vi "周期设置_总磷总氮.vi"() -> ()   [LabVIEW 2016, in "斯坦道氨氮.lvlib"]
uses:
  <vilib>/Utility/miscctls.llb/LVPointTypeDef.ctl
  <vilib>/Utility/config.llb/NI_LVConfig.lvlib
panel:
  in  "运行周期":T1={"运行模式"=enum."维护模式", "质控频次"=enum."关闭", "空白核查时间"=2, "跨度核查时间"=6, "24H周期设置"=[]} {"跨度核查时间" items=["00H", "01H", "02H", "03H", "04H", "05H", "06H", "07H", "08H", "09H", "10H", "11H", "12H", "13H", "14H", "15H", "16H", "17H", "18H", "19H", "20H", "21H", "22H", "23H", "关闭"]; "空白核查时间" items=["00H", "01H", "02H", "03H", "04H", "05H", "06H", "07H", "08H", "09H", "10H", "11H", "12H", "13H", "14H", "15H", "16H", "17H", "18H", "19H", "20H", "21H", "22H", "23H", "关闭"]}
  # "运行模式："
  # "质控频次："
  # "零点核查时间："
  # "跨度核查时间："
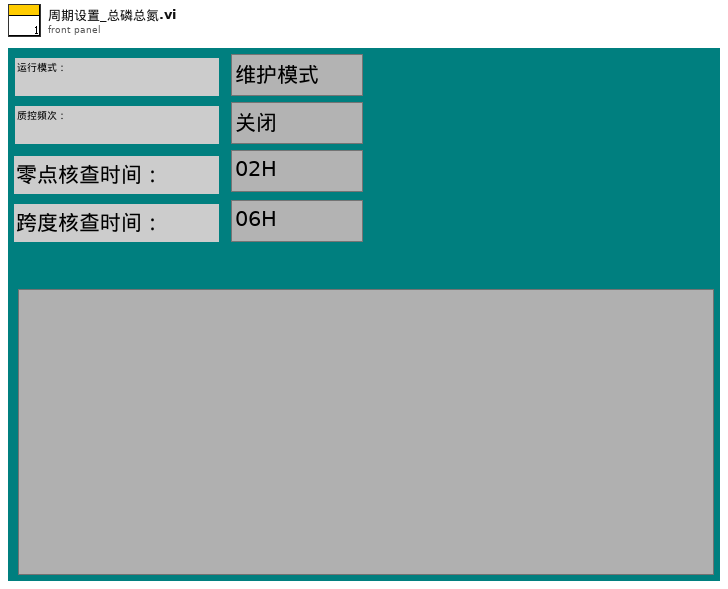
[diagram p1: front panel]
types:
  T1 = cluster{"运行模式":enum16{"维护模式", "常规模式", "应急模式", "质控模式"}, "质控频次":enum16{"关闭", "每天", "星期一", "星期二", "星期三", "星期四", "星期五", "星期六", "星期日"}, "空白核查时间":u16, "跨度核查时间":u16, "24H周期设置":bool[]}
  T2 = typedef "LVPointTypeDef.ctl" = cluster{"Horizontal":i16, "Vertical":i16}
  T3 = enum16{"启动测量", "标样核查", "零点核查", "跨度核查", "空白测试", "平行样测试", "加标回收", "空白校准", "标样校准", "初始化（清洗）", "停止测试", "仪器重启", "校时", "模式设置", "测量间隔设置"}
  T4 = cluster{"系统时间":timestamp, "工作状态":enum16{"空闲", "水样测试", "标样核查", "零点核查", "跨度核查", "空白测试", "平行样测试", "加标回收", "空白校准", "标样校准", "初始化（清洗）"}, "测量模式":enum16{"待机", "连续模式", "周期模式", "定点模式", "受控模式", "手动模式"}, "告警代码":u16, "故障代码":u16, "日志代码":u16, "软件版本":u16, "F0":sgl, "F1":sgl, "F2":sgl, "F3":sgl, "T":sgl, "H":sgl, "id":u16, "flowid":u16, "量程":u16, "总磷控温温度1":sgl, "营养盐控温温度2":sgl, "ADC":sgl}
  T5 = enum16{"关闭", "每天", "星期一", "星期二", "星期三", "星期四", "星期五", "星期六", "星期日"}
  T6 = typedef "LVDateTimeRec.ctl" = cluster{"秒数的小数部分":dbl, "秒":i32, "分":i32, "时":i32, "日":i32, "月":i32, "年":i32, "天数（周）":i32, "天数（年）":i32, "DST":i32}
  T7 = enum32{"Bad", "Idle", "Run top level", "Running"}
  T8 = typedef "NI_LVConfig.lvlib/Config Data RefNum.ctl" = refnum<k1>
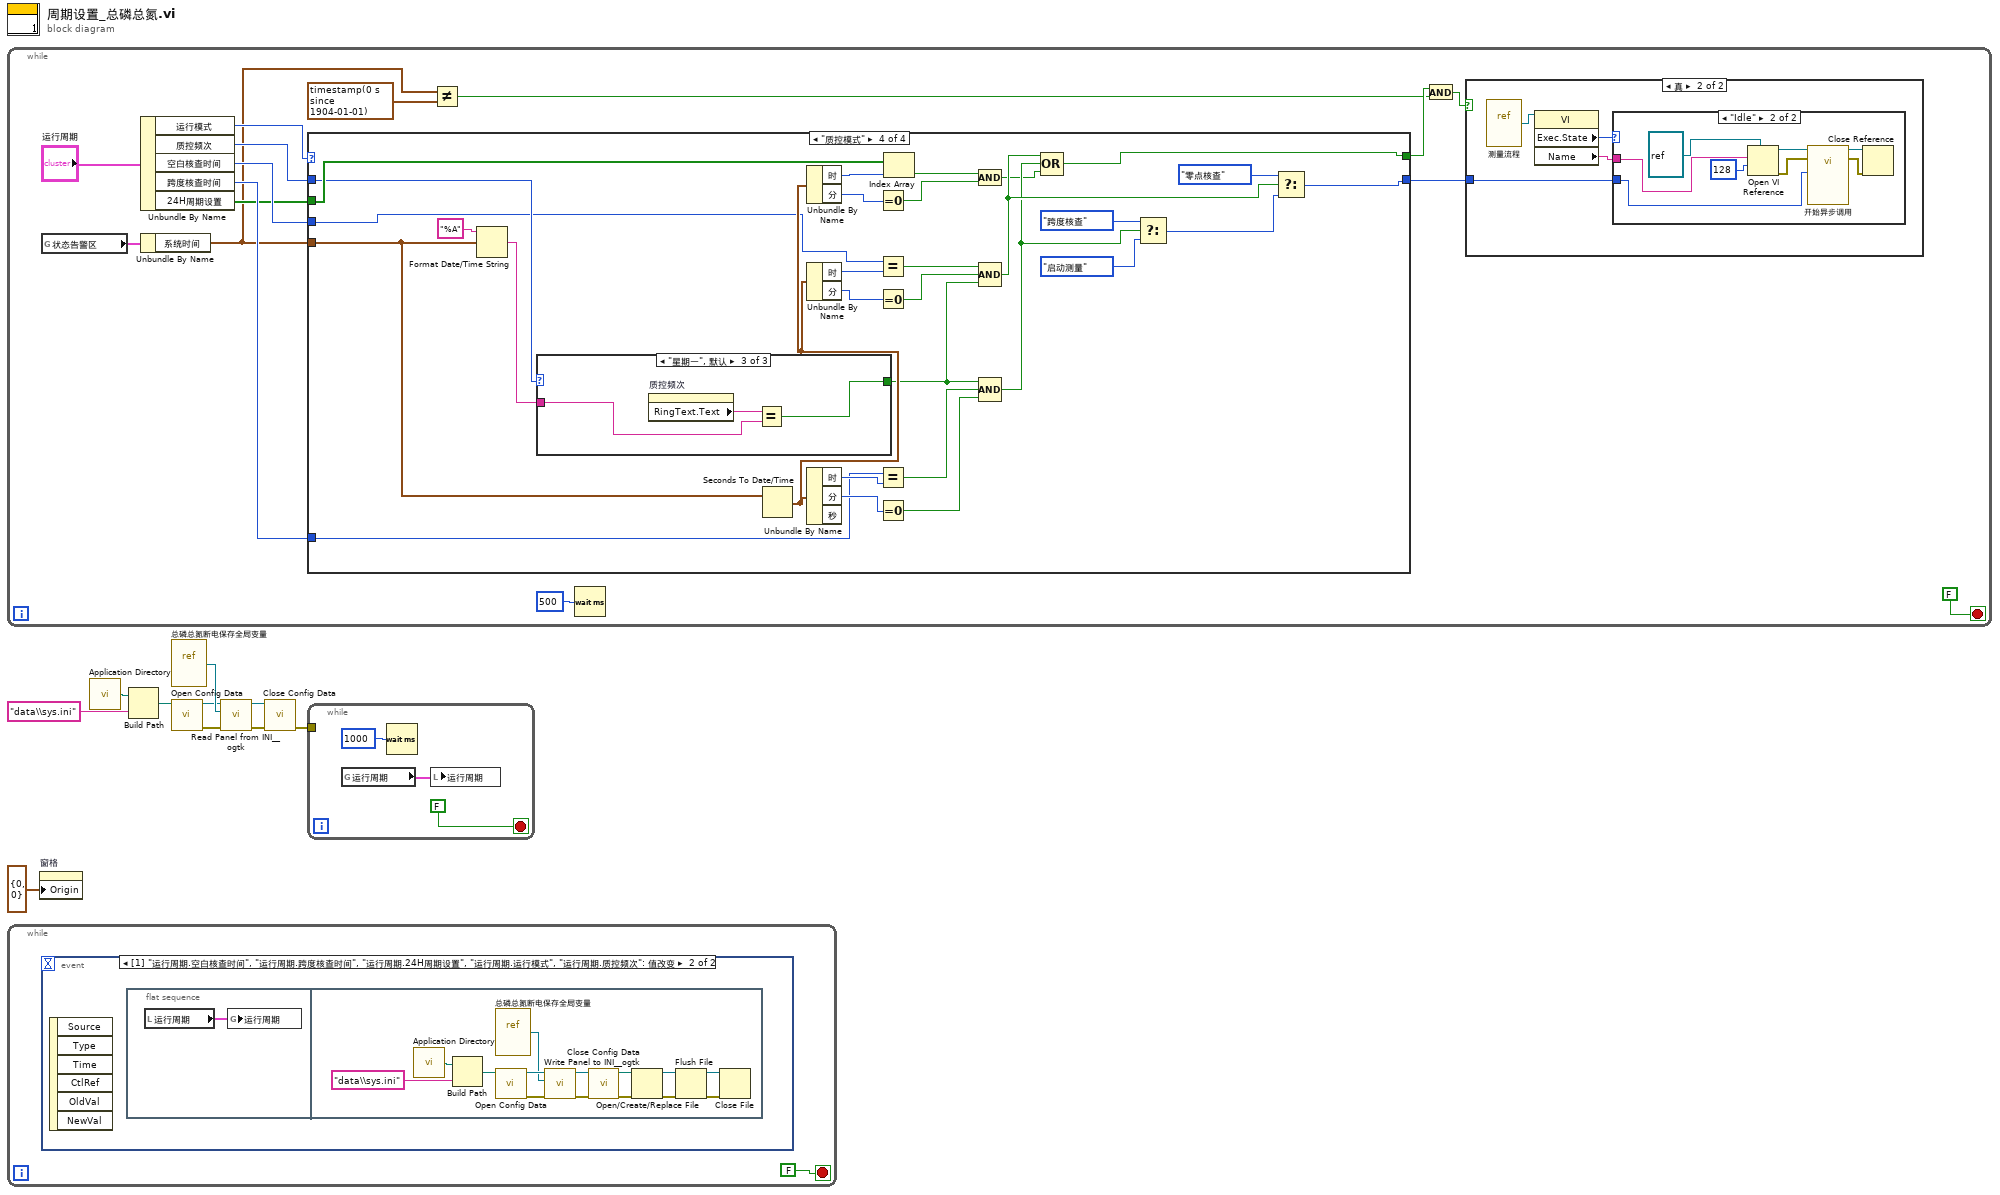
[diagram p0: block diagram]
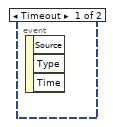
[diagram p2: hidden frame]
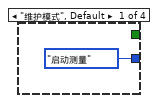
[diagram p5: hidden frame]
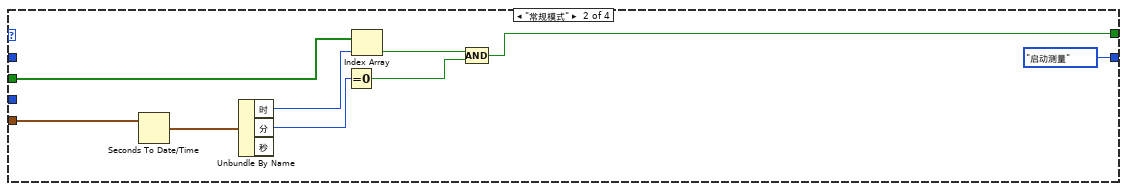
[diagram p6: hidden frame]
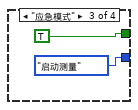
[diagram p7: hidden frame]
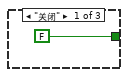
[diagram p8: hidden frame]
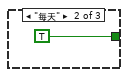
[diagram p9: hidden frame]
diagram:
  n1 = while {
    stop <- FALSE stop-if-true
    n2 = global read "VAR总磷总氮全局变量.vi" "状态告警区"() -> (w15:T4)
    n3 = Unbundle By Name("运行周期") -> ("运行模式"=w22:enum16{"维护模式", "常规模式", "应急模式", "质控模式"}, "质控频次"=w21:T5, "空白核查时间"=w20:u16, "跨度核查时间"=w19:u16, "24H周期设置"=w18:bool[])
    n4 = Unbundle By Name(w15) -> ("系统时间"=w14:timestamp)
    n5 = case shown="\"质控模式\"" w22 {
      tunnel: w14 -> [_ w47 _ w79]
      tunnel: w18 -> [_ w44 _ w76]
      tunnel: [_ w40 TRUE w62] -> w17
      tunnel: [T3."启动测量" ("控制命令") T3."启动测量" ("控制命令") T3."启动测量" ("控制命令") w58] -> w16
      tunnel: w21 -> [_ _ _ w55]
      tunnel: w20 -> [_ _ _ w54]
      tunnel: w19 -> [_ _ _ w53]
      frame "维护模式", Default {
      }
      frame "常规模式" {
        n6 = Seconds To Date/Time(time stamp (now)=w47) -> (date time rec=w46:T6)  [unwired: 1 in]
        n7 = Unbundle By Name(w46) -> ("时"=w45:i32, "分"=w43:i32)  [unwired: 1 out]
        n8 = Equal To 0?(x=w43) -> (x = 0?=w41:bool)
        n9 = Index Array(array=w44, index=w45) -> (element=w42:bool)
        n10 = Compound Arithmetic op=AND ("复合运算")(w42, w41) -> (w40:bool)
      }
      frame "应急模式" {
      }
      frame "质控模式" {
        n11 = Format Date/Time String(time format string (%c)="%A" ("时间格式字符串(%c)"), seconds (now)=w79) -> (date/time string=w77:string)  [unwired: 1 in]
        n12 = case shown="\"星期一\", 默认" w55 {
          tunnel: w77 -> [_ _ w83]
          tunnel: [FALSE TRUE w82] -> w56
          frame "关闭" {
          }
          frame "每天" {
          }
          frame "星期一", Default {
            n13 = property on="质控频次" class="Enum (严格)"() -> ("RingText.Text"=w84:string)  [unwired: 2 in, 2 out]
            n14 = Equal?(x=w84, y=w83) -> (x = y?=w82:bool)
          }
        }
        n15 = Seconds To Date/Time(time stamp (now)=w79) -> (date time rec=w65:T6)  [unwired: 1 in]
        n16 = Unbundle By Name(w65) -> ("时"=w75:i32, "分"=w73:i32)
        n17 = Unbundle By Name(w65) -> ("时"=w71:i32, "分"=w70:i32)
        n18 = Unbundle By Name(w65) -> ("时"=w66:i32, "分"=w67:i32)  [unwired: 1 out]
        n19 = Equal To 0?(x=w73) -> (x = 0?=w72:bool)
        n20 = Equal?(x=w54, y=w71) -> (x = y?=w69:bool)
        n21 = Equal To 0?(x=w70) -> (x = 0?=w68:bool)
        n22 = Equal?(x=w53, y=w66) -> (x = y?=w64:bool)
        n23 = Equal To 0?(x=w67) -> (x = 0?=w63:bool)
        n24 = Index Array(array=w76, index=w75) -> (element=w74:bool)
        n25 = Compound Arithmetic op=AND ("复合运算")(w74, w72) -> (w57:bool)
        n26 = Compound Arithmetic op=AND ("复合运算")(w69, w68, w56) -> (w61:bool)
        n27 = Compound Arithmetic op=AND ("复合运算")(w56, w64, w63) -> (w60:bool)
        n28 = Compound Arithmetic op=OR ("复合运算")(w61, w60, w57) -> (w62:bool)
        n29 = Select(t=T3."跨度核查" ("控制命令"), s=w60, f=T3."启动测量" ("控制命令")) -> (s? t:f=w59:T3)
        n30 = Select(t=T3."零点核查" ("控制命令"), s=w61, f=w59) -> (s? t:f=w58:T3)
      }
    }
    n31 = Not Equal?(x=w14, y=timestamp(0 s since 1904-01-01)) -> (x != y?=w11:bool)
    n32 = Wait (ms)(milliseconds to wait=u32 500 ("等待时间（毫秒）")) -> ()  [unwired: 1 out]
    n33 = And(x=w17, y=w11) -> (x .and. y?=w12:bool)
    n34 = case shown="真" w12 {
      tunnel: w16 -> [_ w27]
      frame False {
      }
      frame True {
        n35 = vi-ref "测量流程.vi"() -> (w28:refnum<vi>)
        n36 = property class="VI"(reference=w28) -> ("Exec.State"=w26:T7, "Name"=w29:string)  [unwired: 1 in, 2 out]
        n37 = case shown="\"Idle\"" w26 {
          tunnel: w29 -> [_ w33]
          tunnel: w27 -> [_ w30]
          frame "Bad", Default {
          }
          frame "Idle" {
            n38 = Open VI Reference(type specifier VI Refnum (for type only)=refnum<vi> refnum, vi path=w33, options=128 ("选项")) -> (vi reference=w34:refnum<vi>, error out=w35:errorcluster)  [unwired: 3 in]
            n39 = call-by-ref "开始异步调用"(reference=w34, error in=w35, "控制命令"=w30) -> (reference out=w36:refnum<vi>, error out=w37:errorcluster)  [unwired: 11 in]
            n40 = Close Reference(reference=w36, error in (no error)=w37) -> ()  [unwired: 1 out]
          }
        }
      }
    }
  }
  n41 = while {
    stop <- FALSE stop-if-true
    n42 = event shown="[1] \"运行周期.空白核查时间\", \"运行周期.跨度核查时间\", \"运行周期.24H周期设置\", \"运行周期.运行模式\", \"运行周期.质控频次\": 值改变" {
      selector: _ -> [_ _]
      dyn-events: _ -> [_ _]
      timeout: _ -> [_ _]
      event Timeout {
        n43 = event-data() -> ()  [unwired: 1 in, 3 out]
      }
      event "运行周期.空白核查时间", "运行周期.跨度核查时间", "运行周期.24H周期设置", "运行周期.运行模式", "运行周期.质控频次": Value Change {
        n44 = event-data() -> ()  [unwired: 1 in, 6 out]
        n45 = flat-sequence {
          frame #0 {
            n46 = local read "运行周期"() -> (w86:T1)
            n47 = global write "总磷总氮断电保存全局变量.vi" "运行周期"(w86) -> ()
          }
          frame #1 {
            n48 = call <vilib>:"Application Directory.vi"() -> ("Application Directory"=w100:path)
            n49 = Build Path(base path=w100, name or relative path="data\\sys.ini" ("名称或相对路径")) -> (appended path=w98:path)
            n50 = vi-ref "总磷总氮断电保存全局变量.vi"() -> (w96:refnum<vi>)
            n51 = call <vilib>:"Open Config Data.vi"("configuration file path"=w98) -> ("error out"=w94:errorcluster, "refnum"=w97:T8)  [unwired: 8 in, 1 out]
            n52 = call <userlib>:"Write Panel to INI__ogtk.vi"("error in (no error)"=w94, "VI ref"=w96, "refnum"=w97) -> ("error out"=w93:errorcluster, "refnum out"=w95:T8)  [unwired: 7 in]
            n53 = call <vilib>:"Close Config Data.vi"("error in (no error)"=w93, "refnum"=w95) -> ("error out"=w88:errorcluster, "file path"=w87:path)  [unwired: 8 in]
            n54 = Open/Create/Replace File(file path (use dialog)=w87, error in=w88) -> (refnum out=w91:refnum<file>, error out=w92:errorcluster)  [unwired: 4 in, 1 out]
            n55 = Flush File(refnum=w91, error in=w92) -> (refnum out=w90:refnum<file>, error out=w89:errorcluster)
            n56 = Close File(refnum=w90, error in=w89) -> ()  [unwired: 2 out]
          }
        }
      }
    }
  }
  n57 = property on="窗格" class="Pane"("Origin"=T2 {"Horizontal"=0, "Vertical"=0} ("原点")) -> ()  [unwired: 2 in, 2 out]
  n58 = call <vilib>:"Application Directory.vi"() -> ("Application Directory"=w3:path)
  n59 = Build Path(base path=w3, name or relative path="data\\sys.ini" ("名称或相对路径")) -> (appended path=w5:path)
  n60 = vi-ref "总磷总氮断电保存全局变量.vi"() -> (w7:refnum<vi>)
  n61 = call <vilib>:"Open Config Data.vi"("configuration file path"=w5) -> ("error out"=w9:errorcluster, "refnum"=w6:T8)  [unwired: 8 in, 1 out]
  n62 = call <userlib>:"Read Panel from INI__ogtk.vi"("error in (no error)"=w9, "VI ref"=w7, "refnum"=w6) -> ("error out"=w10:errorcluster, "refnum out"=w8:T8)  [unwired: 7 in]
  n63 = call <vilib>:"Close Config Data.vi"("error in (no error)"=w10, "refnum"=w8) -> ("error out"=w2:errorcluster)  [unwired: 8 in, 1 out]
  n64 = while {
    tunnel: w2 -> [_]
    stop <- FALSE stop-if-true
    n65 = global read "总磷总氮断电保存全局变量.vi" "运行周期"() -> (w101:T1)
    n66 = Wait (ms)(milliseconds to wait=u32 1000 ("等待时间（毫秒）")) -> ()  [unwired: 1 out]
    n67 = local write "运行周期"(w101) -> ()
  }
